vi "Autosampler Status Update.vi"(8 "error in (no error)":errorcluster, 10 "Autosampler Status":T1, 11 "Main Window in":refnum<class "Main Window.lvclass">) -> (0 "error out":errorcluster, 3 "Main Window out":refnum<class "Main Window.lvclass">)   [LabVIEW 2023, in "Main Window.lvlib" / "Main Window.lvclass"]
uses:
  Main Window.lvclass
  Main Window.lvclass/Main Window.ctl
  Hardware/Autosampler/Autosampler Status.ctl
  Hardware/Autosampler/Autosampler.lvlib
  Hardware/Autosampler/Autosampler State.ctl
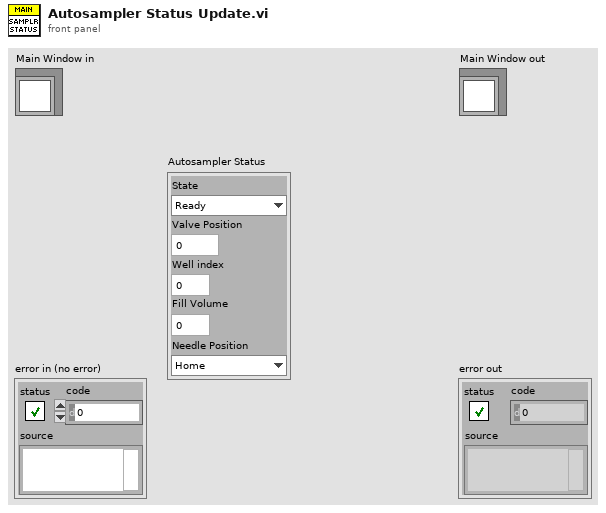
[diagram p1: front panel]
types:
  T1 = typedef "Autosampler.lvlib/Autosampler Status.ctl" = cluster{"State":T2, "Valve Position":u16, "Well index":u16, "Fill Volume":u16, "Needle Position":enum16{"Home", "Well", "Wash Port"}}
  T2 = typedef "Autosampler.lvlib/Autosampler State.ctl" = enum16{"Ready", "Injection", "Washing", "Shaking", "Getting Ready", "Error"}
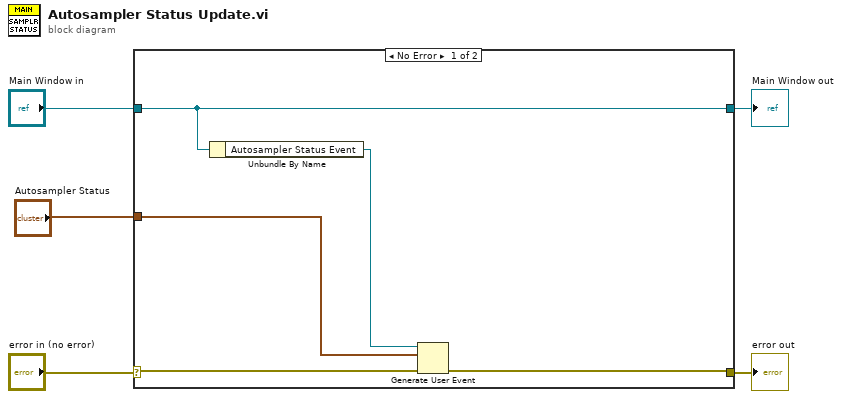
[diagram p0: block diagram]
diagram:
  n1 = case shown="No Error" "error in (no error)" {
    selector: "error in (no error)" -> [w10 w12]
    tunnel: [w9 w12] -> w4
    tunnel: [w8 w11] -> w2
    tunnel: "Main Window in" -> [w8 w11]
    tunnel: "Autosampler Status" -> [w6 _]
    frame No Error {
      n2 = Unbundle By Name(w8) -> ("Autosampler Status Event"=w7:refnum<user-event>)
      n3 = Generate User Event(user event=w7, event data cluster=w6, error in=w10) -> (error out=w9:errorcluster)  [unwired: 1 in, 1 out]
    }
    frame Error {
    }
  }
  "error out" <- w4
  "Main Window out" <- w2
